vi "Robot Drive Manual - Tank.vi"(0 "Left Side Value":dbl, 2 "Right Side Bias":dbl, 3 "Left Side Bias":dbl, 5 "Gear Shift Data":T1, 7 "RobotDriveDevRef":T2, 9 "Right Side Value":dbl, 12 "Gear Shift Throttle Limit":dbl, 13 "High Gear Multiplier":dbl, 14 "Low Gear Multiplier":dbl) -> (4 "Motor Values":dbl[](array[numeric]))   [LabVIEW 2016]
uses:
  <vilib>/Rock Robotics/WPI/RobotDrive/WPI_RobotDriveDevRef.ctl
  <vilib>/Rock Robotics/WPI/MotorControl/WPI_MotorControlDeviceRef.ctl
  <vilib>/Rock Robotics/WPI/MotorControl/WPI_MotorControlType.ctl
  <vilib>/Rock Robotics/SystemInterfaces/DIO/FPGA_DIOPWMChannel.ctl
  <vilib>/Rock Robotics/WPI/PWM/WPI_PWMDeadband.ctl
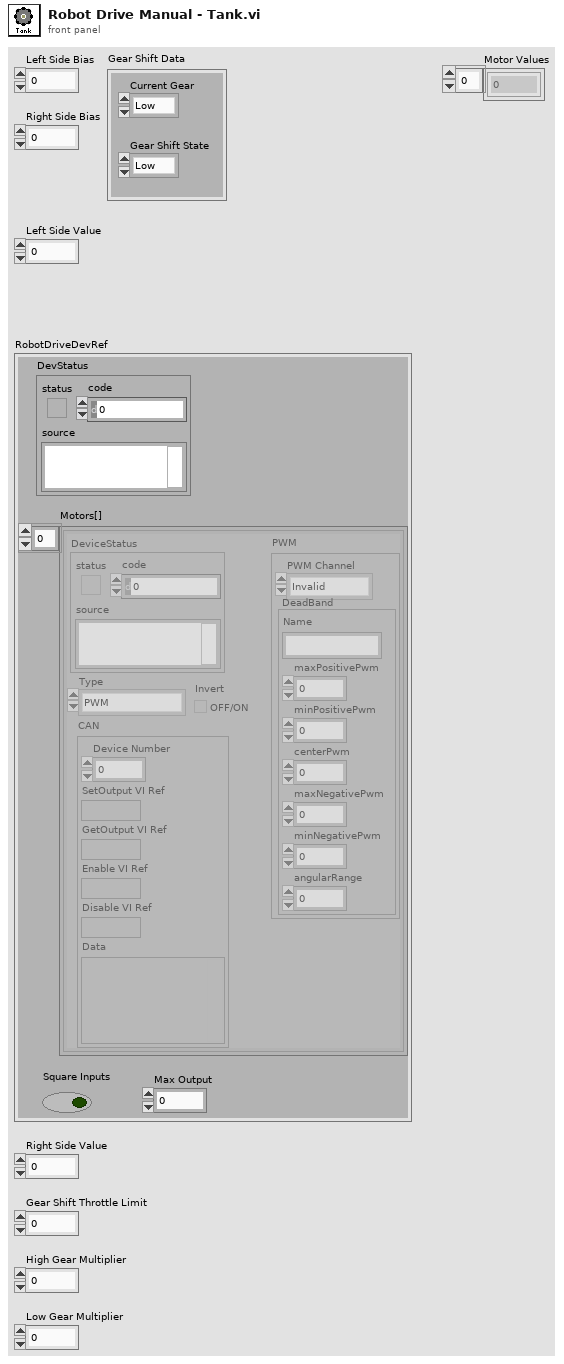
[diagram p1: front panel]
types:
  T1 = cluster{"Current Gear":enum16{"Low", "High"}, "Gear Shift State":enum16{"Low", "Shifting", "High"}}
  T2 = typedef "WPI_RobotDriveDevRef.ctl" = cluster{"DevStatus":errorcluster, "Motors[]":T3[], "Square Inputs":bool, "Max Output":dbl}
  T3 = typedef "WPI_MotorControlDeviceRef.ctl" = cluster{"DeviceStatus":errorcluster, "Type":T4, "PWM":cluster{"PWM Channel":T5, "DeadBand":T6}, "CAN":cluster{"Device Number":u8, "SetOutput VI Ref":variant, "GetOutput VI Ref":variant, "Enable VI Ref":variant, "Disable VI Ref":variant, "Data":variant}, "Invert":bool}
  T4 = typedef "WPI_MotorControlType.ctl" = enum16{"PWM", "CAN"}
  T5 = typedef "FPGA_DIOPWMChannel.ctl" = enum8{"PWM 0", "PWM 1", "PWM 2", "PWM 3", "PWM 4", "PWM 5", "PWM 6", "PWM 7", "PWM 8", "PWM 9", "PWM MXP 0", "PWM MXP 1", "PWM MXP 2", "PWM MXP 3", "PWM MXP 4", "PWM MXP 5", "PWM MXP 6", "PWM MXP 7", "PWM MXP 8", "PWM MXP 9", "Invalid"}
  T6 = typedef "WPI_PWMDeadband.ctl" = cluster{"Name":string, "maxPositivePwm":i32, "minPositivePwm":i32, "centerPwm":i32, "maxNegativePwm":i32, "minNegativePwm":i32, "angularRange":u16}
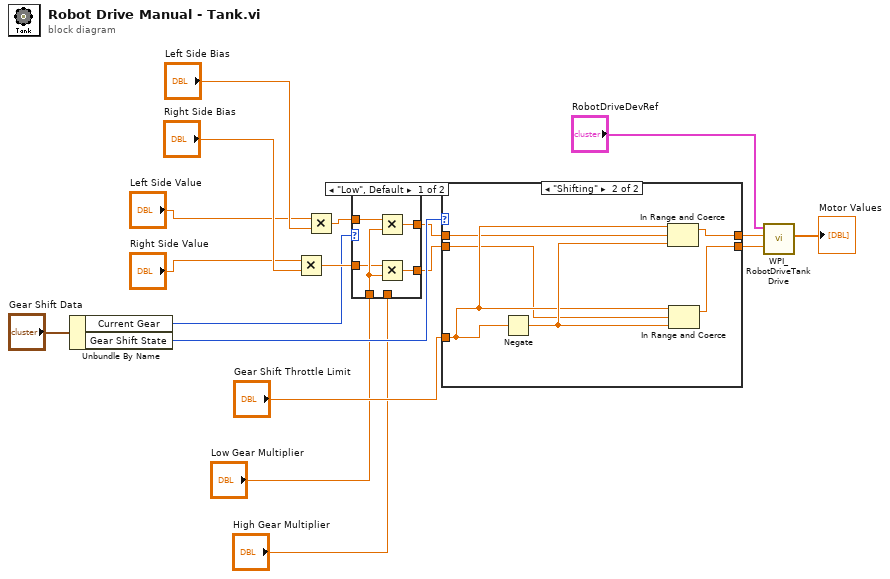
[diagram p0: block diagram]
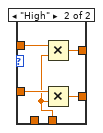
[diagram p2: hidden frame]
diagram:
  n1 = Unbundle By Name("Gear Shift Data") -> ("Current Gear"=w9:enum16{"Low", "High"}, "Gear Shift State"=w10:enum16{"Low", "Shifting", "High"})
  n2 = Multiply(x="Right Side Value", y="Right Side Bias") -> (x*y=w18:dbl)
  n3 = Multiply(x="Left Side Value", y="Left Side Bias") -> (x*y=w17:dbl)
  n4 = case shown="\"Low\", Default" w9 {
    tunnel: w17 -> [w22 w28]
    tunnel: w18 -> [w21 w27]
    tunnel: [w19 w26] -> w5
    tunnel: [w20 w25] -> w6
    tunnel: "Low Gear Multiplier" -> [w23 _]
    tunnel: "High Gear Multiplier" -> [_ w24]
    frame "Low", Default {
      n5 = Multiply(x=w22, y=w23) -> (x*y=w20:dbl)
      n6 = Multiply(x=w21, y=w23) -> (x*y=w19:dbl)
    }
    frame "High" {
      n7 = Multiply(x=w28, y=w24) -> (x*y=w25:dbl)
      n8 = Multiply(x=w27, y=w24) -> (x*y=w26:dbl)
    }
  }
  n9 = case shown="\"Shifting\"" w10 {
    tunnel: [w30 w32] -> w4
    tunnel: w6 -> [w30 w34]
    tunnel: [w29 w31] -> w3
    tunnel: w5 -> [w29 w33]
    tunnel: "Gear Shift Throttle Limit" -> [_ w35]
    frame Default {
    }
    frame "Shifting" {
      n10 = Negate(x=w35) -> (-x=w36:dbl)
      n11 = In Range and Coerce(upper limit=w35, x=w34, lower limit=w36) -> (coerced(x)=w32:dbl)  [unwired: 1 out]
      n12 = In Range and Coerce(upper limit=w35, x=w33, lower limit=w36) -> (coerced(x)=w31:dbl)  [unwired: 1 out]
    }
  }
  n13 = call <vilib>:"WPI_RobotDriveTankDrive.vi"("Right axis value"=w3, "Left axis value"=w4, "RobotDriveDevRef"="RobotDriveDevRef") -> ("Motor Values"=→"Motor Values":dbl[])  [unwired: 6 in, 2 out]
